vi "WSVCAP SHL Host LL Interface Core.vi"(0 "Message In":string, 11 "error in":errorcluster, 12 "Log (T)":bool=TRUE, 13 "Function":T5, 14 "FPGA":T1) -> (3 "System":T2={"Settings"={"I2C Slave Address"=144, "I2C Clock Rate (Hz)"=20.0, "SRL Clock Rate (Hz)"=50000.0, "Simulate FPGA"=TRUE, "C1 Cap DAC Default"=165, "C2 Cap DAC Default"=165, "C3 Cap DAC Default"=134, "C4 Cap DAC Default"=150, "DAC Out Vref (V)"=0.0}, "FPGA Resource"="", "Online"=FALSE, "I2C Wait Ticks"=0, "SRL Wait Ticks"=0, "FPGA VI Reference (FPGA Mode)"=refnum, "FPGA VI Reference (Sim Mode)"=refnum} {"Settings"."DAC Out Vref (V)" format="%.3f V"; "Settings"."C4 Cap DAC Default" format="0x%02x"; "Settings"."C3 Cap DAC Default" format="0x%02x"; "Settings"."C2 Cap DAC Default" format="0x%02x"; "Settings"."C1 Cap DAC Default" format="0x%02x"; "Settings"."SRL Clock Rate (Hz)" format="%.0f Hz"; "Settings"."I2C Clock Rate (Hz)" format="%.0f Hz"; "Settings"."I2C Slave Address" format="0x%02x"}, 4 "Message Out":string, 15 "error out":errorcluster)   [LabVIEW 2017]
uses:
  Type Defs/WSVCAP SHL Function Enum.ctl
  Type Defs/WSVCAP SHL Core System Cluster.ctl
  Type Defs/WSVCAP SHL I2C Settings Cluster.ctl
  Type Defs/WSVCAP SHL FPGA Ref.ctl
  Type Defs/WSVCAP SHL FPGA Enum.ctl
  user.lib/Utilities/Type Defs/MISC IO Choice Enum.ctl
  Type Defs/WSVCAP SHL Gatekeeper Operation Enum.ctl
  user.lib/Configuration Files/Type Defs/CFG File Operation Enum.ctl
  Type Defs/WSVCAP SHL Top Level Control Enum.ctl
  <vilib>/FPGAPlugInAG/PXI-7813R/niLvFpga_Open_PXI-7813R.vi
  <vilib>/FPGAPlugInAG/PXI-7813R/niLvFpga_Reset_PXI-7813R.vi
  <vilib>/FPGAPlugInAG/PXI-7813R/niLvFpga_Run_PXI-7813R.vi
  <vilib>/FPGAPlugInAG/PXI-7813R/niLvFpga_Abort_PXI-7813R.vi
  <vilib>/FPGAPlugInAG/PXI-7813R/niLvFpga_Close_PXI-7813R.vi
  <vilib>/rvi/interface/nirviOpenFPGA/nirviOpenFPGA.xnode
  FPGA Bitfiles/WSVCAPShell_WiSpryFPGA1_WSVCAPSHLFPGATLT_ffr+nD2N+rA.lvbitx
  <vilib>/rvi/interface/nirviMethod/nirviMethod.xnode
  <vilib>/rvi/interface/nirviCloseFPGA/nirviCloseFPGA.xnode
  Host SRL/Host SRL.lvlib
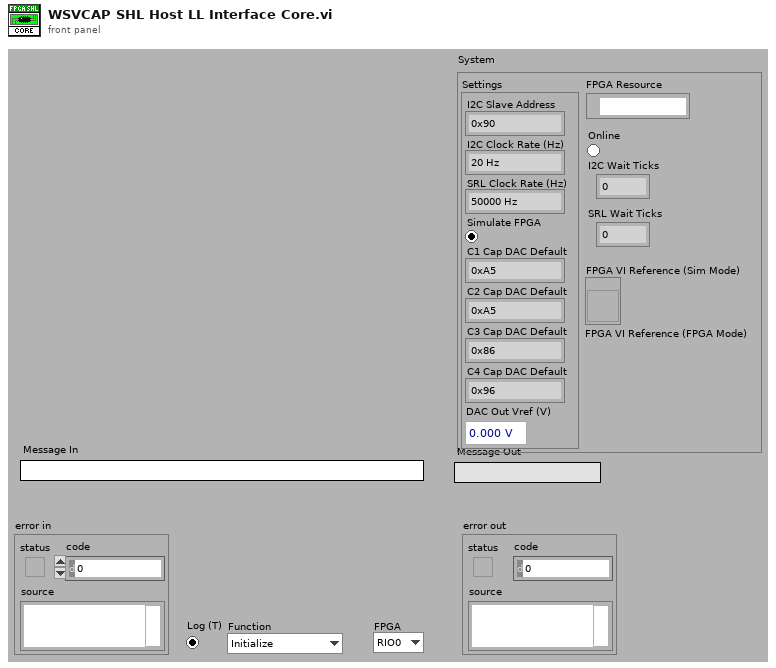
[diagram p1: front panel]
types:
  T1 = typedef "WSVCAP SHL FPGA Enum.ctl" = enum16{"RIO0", "RIO1"}
  T2 = typedef "WSVCAP SHL Core System Cluster.ctl" = cluster{"Settings":T3, "FPGA Resource":tag, "Online":bool, "I2C Wait Ticks":u32, "SRL Wait Ticks":u32, "FPGA VI Reference (FPGA Mode)":T4, "FPGA VI Reference (Sim Mode)":refnum<vi>}
  T3 = typedef "WSVCAP SHL I2C Settings Cluster.ctl" = cluster{"I2C Slave Address":u8, "I2C Clock Rate (Hz)":dbl, "SRL Clock Rate (Hz)":dbl, "Simulate FPGA":bool, "C1 Cap DAC Default":u8, "C2 Cap DAC Default":u8, "C3 Cap DAC Default":u8, "C4 Cap DAC Default":u8, "DAC Out Vref (V)":dbl}
  T4 = typedef "WSVCAP SHL FPGA Ref.ctl" = refnum<k20>
  T5 = typedef "WSVCAP SHL Function Enum.ctl" = enum16{"Initialize", "Configure I2C", "Configure SRL", "Write I2C", "Read I2C", "Write SRL", "Start SRL Cycle", "Stop SRL Cycle", "Get Status", "Close"}
  T6 = typedef "WSVCAP SHL Gatekeeper Operation Enum.ctl" = enum16{"Initialize", "Lock", "Unlock", "Close"}
  T7 = typedef "MISC IO Choice Enum.ctl" = enum16{"Read", "Write"}
  T8 = typedef "CFG File Operation Enum.ctl" = enum16{"Read", "Write", "Copy", "Edit"}
  T9 = enum32{"Invalid", "Standard", "Closed", "Hidden", "Minimized", "Maximized"}
  T10 = typedef "WSVCAP SHL Top Level Control Enum.ctl" = enum16{"Start", "Cmd", "Transaction", "Wait Ticks", "Socket Mask", "UUT Set", "Slave Address", "Sub Address", "Bytes to Write", "Bytes to Read", "Write Data", "Write Flag", "Read Data", "Read Flag", "Ack Read", "Read Status Flag", "Ack Read Status", "Status", "Cycle Count", "Stop Cycle", "Exit"}
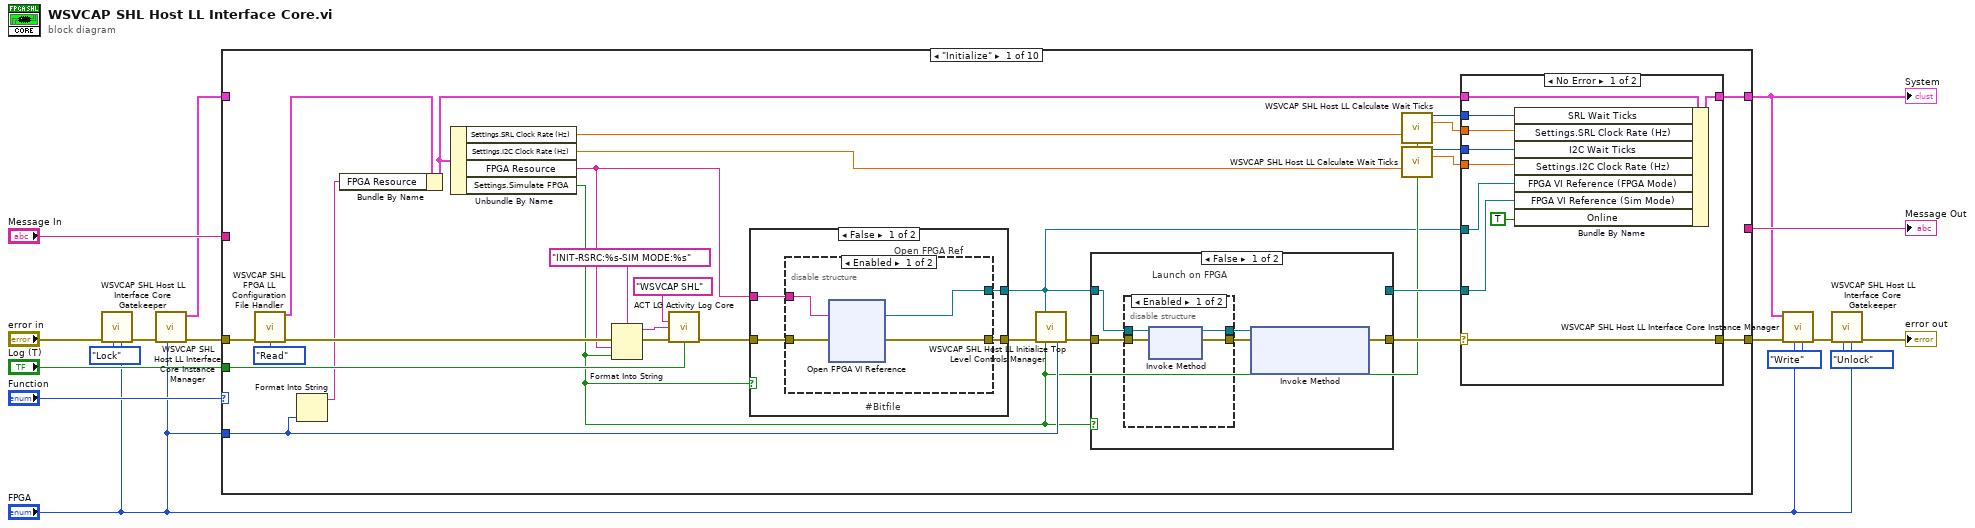
[diagram p0: block diagram]
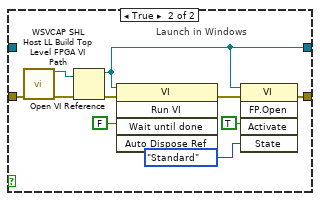
[diagram p5: hidden frame]
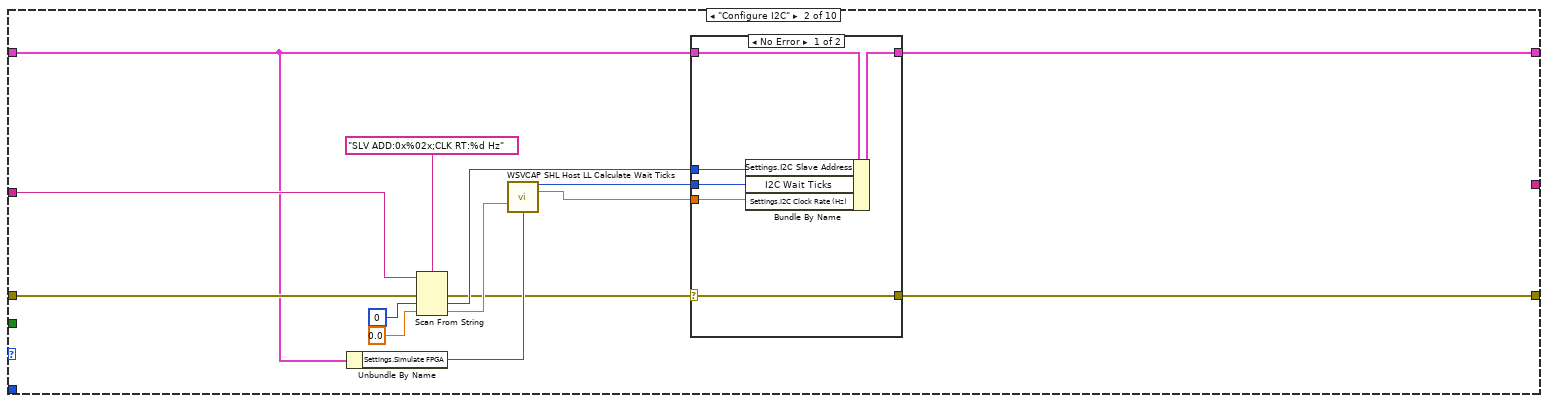
[diagram p7: hidden frame]
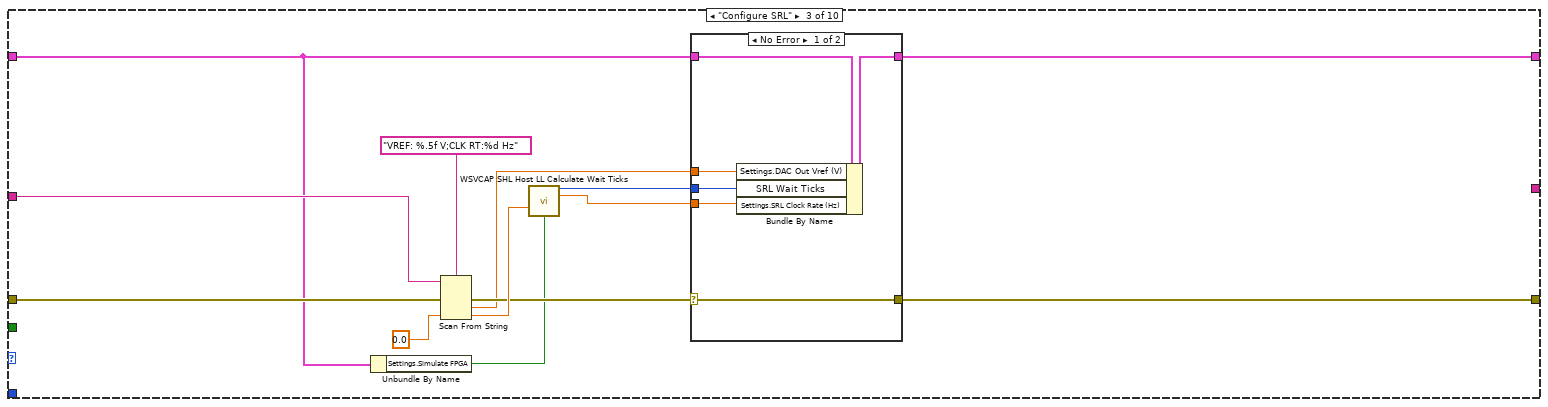
[diagram p9: hidden frame]
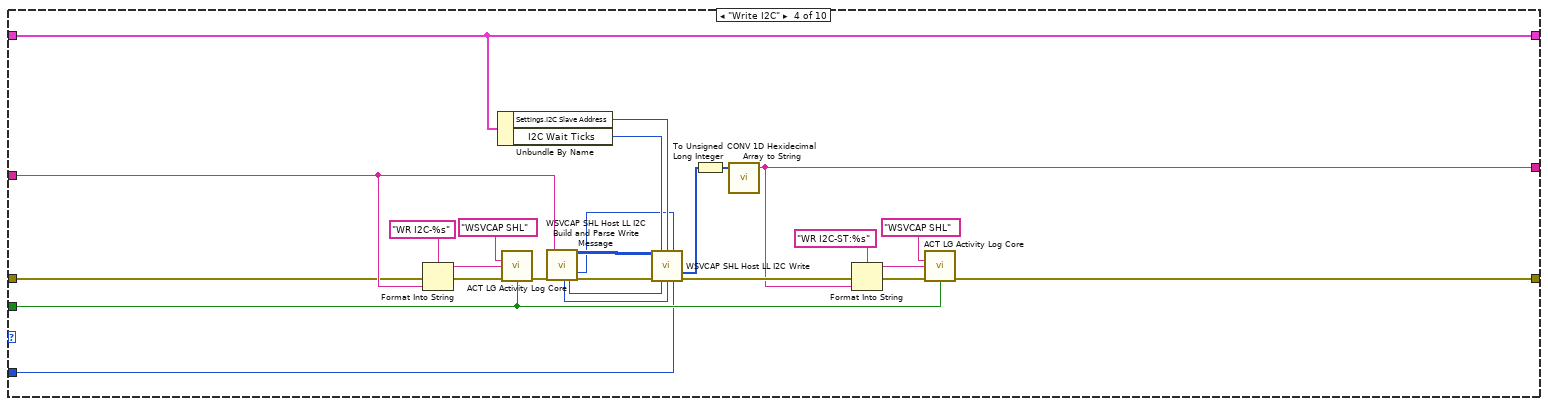
[diagram p11: hidden frame]
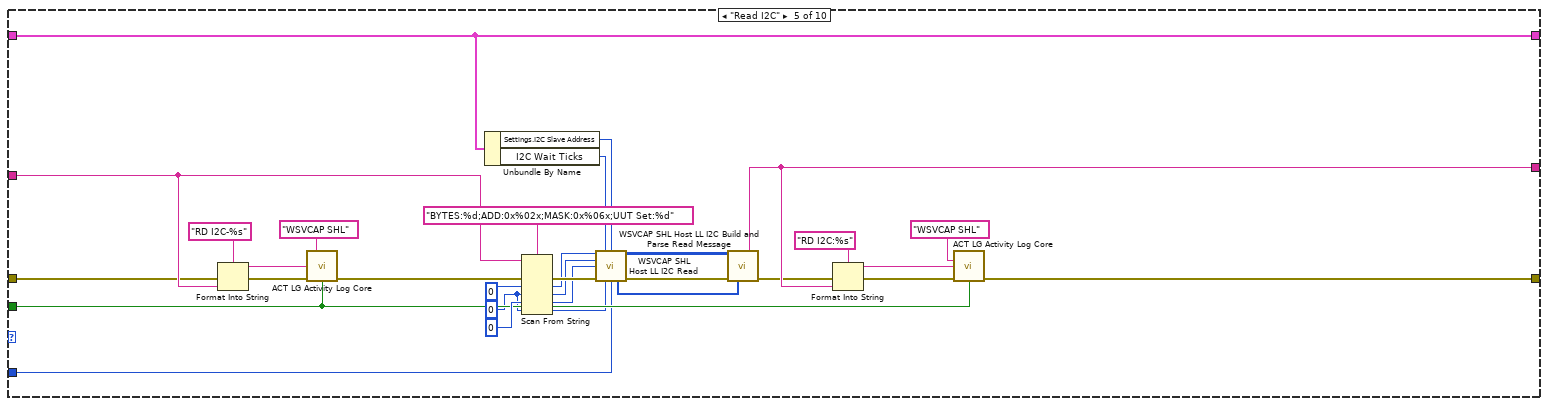
[diagram p12: hidden frame]
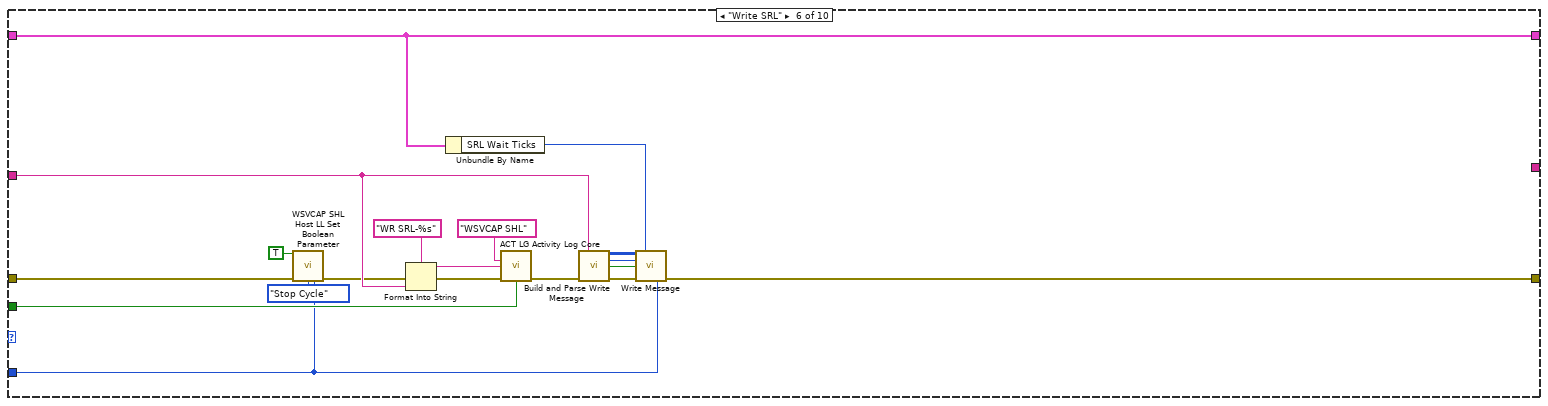
[diagram p13: hidden frame]
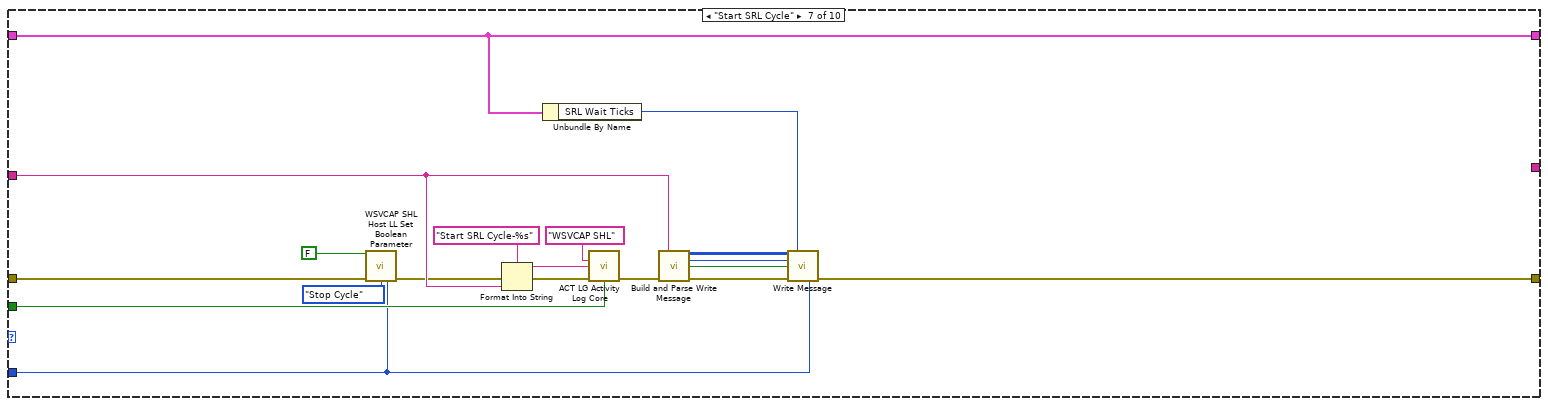
[diagram p14: hidden frame]
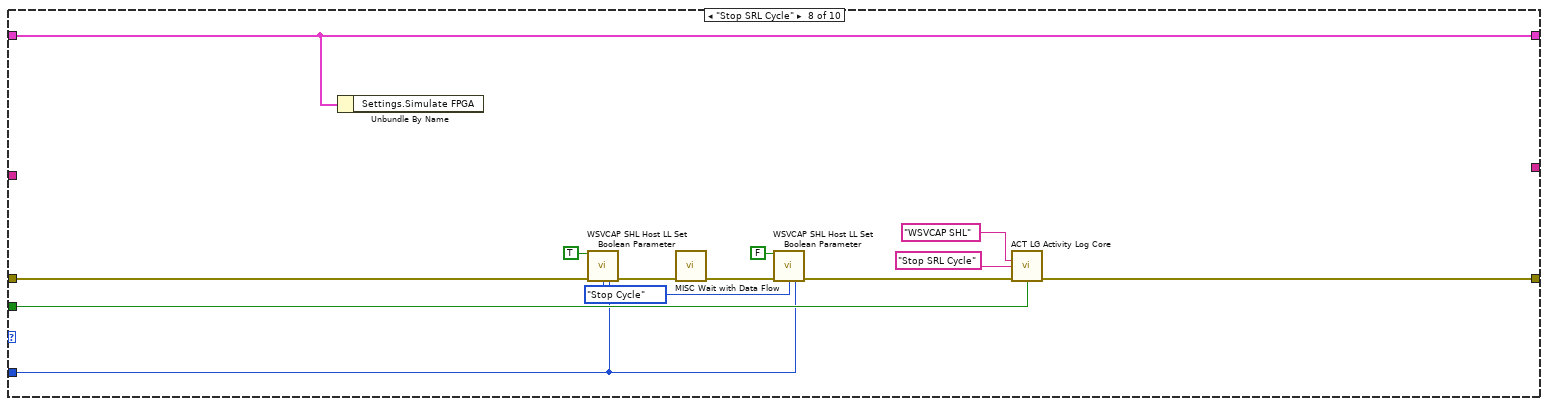
[diagram p15: hidden frame]
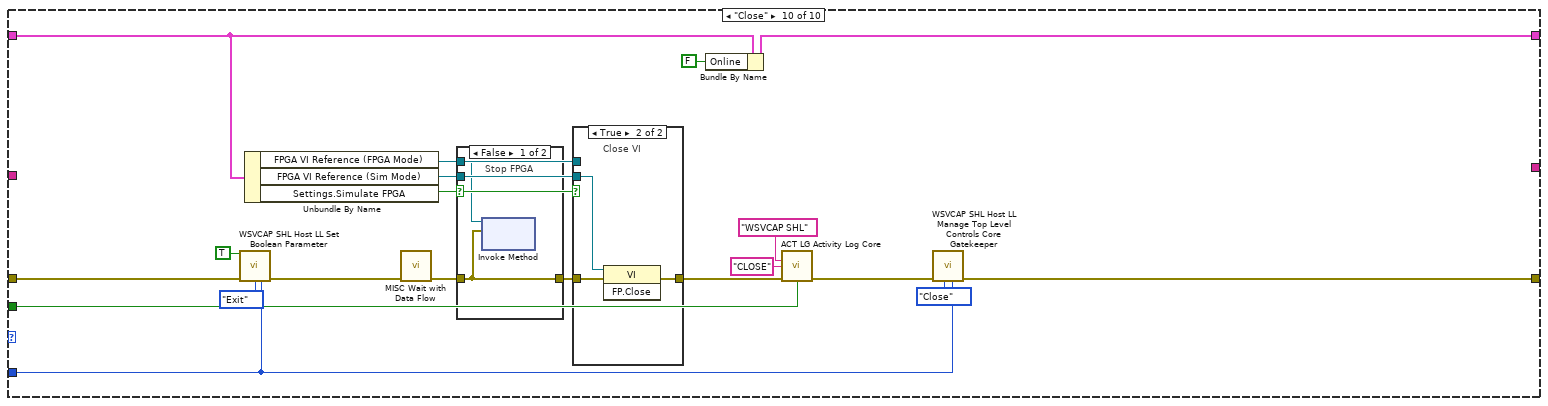
[diagram p17: hidden frame]
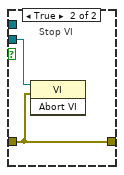
[diagram p18: hidden frame]
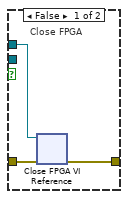
[diagram p19: hidden frame]
diagram:
  n1 = call "WSVCAP SHL Host LL Interface Core Gatekeeper.vi"("FPGA"="FPGA", "Operation"=WSVCAP_SHL_Gatekeeper_Operation_Enum."Lock", "error in (no error)"="error in") -> ("error out"=w4:errorcluster)  [unwired: 8 in]
  n2 = call "WSVCAP SHL Host LL Interface Core Instance Manager.vi"("FPGA"="FPGA", "error in (no error)"=w4) -> ("error out"=w10:errorcluster, "FGPA Interface Out"=w9:T2)  [unwired: 8 in]
  n3 = case shown="\"Initialize\"" "Function" {
    tunnel: w10 -> [w40 w99 w120 w149 w170 w196 w210 w234 w239 w257]
    tunnel: "Message In" -> [_ w98 w119 w150 w171 w199 w218 _ _ _]
    tunnel: [w43 w100 w121 w151 w167 w191 w216 w237 w239 w242] -> w12
    tunnel: [w44 w101 w122 w137 w163 w193 w214 w226 w240 w260] -> w11
    tunnel: w9 -> [_ w94 w117 w137 w163 w193 w214 w226 w240 w250]
    tunnel: [_ _ _ w141 w172 _ _ _ _ _] -> w14
    tunnel: "Log (T)" -> [w33 _ _ w138 w164 w198 w217 w236 _ w253]
    tunnel: "FPGA" -> [w21 _ _ w132 w158 w190 w208 w232 _ w241]
    frame "Initialize" {
      n4 = call "WSVCAP SHL FPGA LL Configuration File Handler.vi"("Error In (no error)"=w40, "Operation"=CFG_File_Operation_Enum."Read") -> ("Object Cluster Out"=w23:T2, "Error Out"=w38:errorcluster)  [unwired: 11 in, 1 out]
      n5 = Format Into String(w21) -> (resulting string=w24:string)  [unwired: 3 in, 1 out]
      n6 = Bundle By Name(cluster=w23, "FPGA Resource"=w24) -> (w22:T2)
      n7 = Unbundle By Name(w22) -> ("Settings.SRL Clock Rate (Hz)"=w31:dbl, "Settings.I2C Clock Rate (Hz)"=w35:dbl, "FPGA Resource"=w28:tag, "Settings.Simulate FPGA"=w20:bool)
      n8 = Format Into String(format string="INIT-RSRC:%s-SIM MODE:%s", error in=w38, w28, w20) -> (resulting string=w39:string, error out=w37:errorcluster)  [unwired: 1 in]
      n9 = call "ACT LG Activity Log Core.vi"("Source"="WSVCAP SHL", "Log Line"=w39, "Error In (no error)"=w37, "Log (T)"=w33) -> ("Error Out"=w27:errorcluster)  [unwired: 10 in, 1 out]
      n10 = case shown="False" w20 {
        tunnel: [w48 w54] -> w19
        tunnel: w27 -> [w47 w54]
        tunnel: [w46 _] -> w17
        tunnel: w28 -> [w45 _]
        frame False {
          # "#Bitfile"
          # "Open FPGA Ref"
          n11 = disable-structure shown="Enabled" {
            disable-tunnel: w47 -> [w52 w53]
            disable-tunnel: [w51 w53] -> w48
            disable-tunnel: [w50 _] -> w46
            disable-tunnel: w45 -> [w49 _]
            frame Enabled {
              n12 = xnode "Open FPGA VI Reference"("error in"=w52, "resource name"=w49) -> ("FPGA VI Reference Out"=w50:T4, "error out"=w51:errorcluster)
            }
            frame Disabled {
            }
          }
        }
        frame True {
          # "Simulate FPGA"
        }
      }
      n13 = call "WSVCAP SHL Host LL Initialize Top Level Controls Manager.vi"("FPGA VI Reference (Init Only)"=w17, "error in (no error)"=w19, "Simulate FPGA (Init Only)"=w20, "FPGA"=w21) -> ("error out"=w18:errorcluster)  [unwired: 11 in]
      n14 = case shown="False" w20 {
        tunnel: w18 -> [w58 w68]
        tunnel: [w57 w71] -> w26
        tunnel: w17 -> [w55 _]
        tunnel: [_ w72] -> w25
        frame False {
          # "Launch on FPGA"
          n15 = disable-structure shown="Enabled" {
            disable-tunnel: [w63 w65] -> w59
            disable-tunnel: w58 -> [w62 w65]
            disable-tunnel: [w61 w64] -> w56
            disable-tunnel: w55 -> [w60 w64]
            frame Enabled {
              n16 = xnode "Invoke Method"("FPGA VI Reference In"=w60, "error in"=w62) -> ("FPGA VI Reference Out"=w61:T4, "error out"=w63:errorcluster)
            }
            frame Disabled {
            }
          }
          n17 = xnode "Invoke Method"("FPGA VI Reference In"=w56, "error in"=w59) -> ("error out"=w57:errorcluster)  [unwired: 1 in, 1 out]
        }
        frame True {
          # "Launch in Windows"
          n18 = call "WSVCAP SHL Host LL Build Top Level FPGA VI Path.vi"("Error In (no error)"=w68) -> ("Top Level FPGA VI Path"=w66:path, "Error Out"=w67:errorcluster)  [unwired: 13 in]
          n19 = Open VI Reference(vi path=w66, error in (no error)=w67) -> (vi reference=w72:refnum<vi>, error out=w75:errorcluster)  [unwired: 4 in]
          n20 = invoke class="VI" method="Run VI"(reference=w72, error in=w75, "Wait until done"=FALSE ("Wait Until Done")) -> (error out=w73:errorcluster)  [unwired: 2 in, 4 out]
          n21 = invoke class="VI" method="FP.Open"(reference=w72, error in=w73, "Activate"=TRUE ("Activate?"), "State"=T9."Standard" ("Front Panel Window:State")) -> (error out=w71:errorcluster)  [unwired: 1 in, 4 out]
        }
      }
      n22 = call "WSVCAP SHL Host LL Calculate Wait Ticks.vi"("Clock Rate (Hz)"=w31, "Simulate FPGA"=w20) -> ("Wait Ticks"=w30:u32, "Actual Rate (Hz)"=w29:dbl)  [unwired: 12 in]
      n23 = call "WSVCAP SHL Host LL Calculate Wait Ticks.vi"("Clock Rate (Hz)"=w35, "Simulate FPGA"=w20) -> ("Wait Ticks"=w32:u32, "Actual Rate (Hz)"=w42:dbl)  [unwired: 12 in]
      n24 = case shown="No Error" w26 {
        selector: w26 -> [w83 w86]
        tunnel: w22 -> [w85 w87]
        tunnel: [w84 w87] -> w44
        tunnel: [w83 w86] -> w43
        tunnel: w42 -> [w82 _]
        tunnel: w32 -> [w81 _]
        tunnel: w30 -> [w80 _]
        tunnel: w29 -> [w79 _]
        tunnel: w17 -> [w77 _]
        tunnel: w25 -> [w76 _]
        frame No Error {
          n25 = Bundle By Name(cluster=w85, "SRL Wait Ticks"=w80, "Settings.SRL Clock Rate (Hz)"=w79, "I2C Wait Ticks"=w81, "Settings.I2C Clock Rate (Hz)"=w82, "FPGA VI Reference (FPGA Mode)"=w77, "FPGA VI Reference (Sim Mode)"=w76, "Online"=TRUE) -> (w84:T2)
        }
        frame Error {
        }
      }
    }
    frame "Configure I2C" {
      n26 = Unbundle By Name(w94) -> ("Settings.Simulate FPGA"=w93:bool)
      n27 = Scan From String(format string="SLV ADD:0x%02x;CLK RT:%d Hz", input string=w98, error in=w99, default 1=u8 0 ("I2C_Slave Address"), default 2=0.0 ("Clock Rate (Hz)")) -> (error out=w88:errorcluster, output 1=w95:u8, output 2=w91:dbl)  [unwired: 1 in, 2 out]
      n28 = call "WSVCAP SHL Host LL Calculate Wait Ticks.vi"("Clock Rate (Hz)"=w91, "Simulate FPGA"=w93) -> ("Wait Ticks"=w89:u32, "Actual Rate (Hz)"=w90:dbl)  [unwired: 12 in]
      n29 = case shown="No Error" w88 {
        selector: w88 -> [w105 w108]
        tunnel: w94 -> [w107 w109]
        tunnel: [w106 w109] -> w101
        tunnel: [w105 w108] -> w100
        tunnel: w95 -> [w104 _]
        tunnel: w90 -> [w103 _]
        tunnel: w89 -> [w102 _]
        frame No Error {
          n30 = Bundle By Name(cluster=w107, "Settings.I2C Slave Address"=w104, "I2C Wait Ticks"=w102, "Settings.I2C Clock Rate (Hz)"=w103) -> (w106:T2)
        }
        frame Error {
        }
      }
    }
    frame "Configure SRL" {
      n31 = Unbundle By Name(w117) -> ("Settings.Simulate FPGA"=w111:bool)
      n32 = Scan From String(format string="VREF: %.5f V;CLK RT:%d Hz", input string=w119, error in=w120, default 2=0.0 ("Clock Rate (Hz)")) -> (error out=w112:errorcluster, output 1=w110:dbl, output 2=w115:dbl)  [unwired: 2 in, 2 out]
      n33 = call "WSVCAP SHL Host LL Calculate Wait Ticks.vi"("Clock Rate (Hz)"=w115, "Simulate FPGA"=w111) -> ("Wait Ticks"=w114:u32, "Actual Rate (Hz)"=w113:dbl)  [unwired: 12 in]
      n34 = case shown="No Error" w112 {
        selector: w112 -> [w126 w129]
        tunnel: w117 -> [w128 w130]
        tunnel: [w127 w130] -> w122
        tunnel: [w126 w129] -> w121
        tunnel: w113 -> [w125 _]
        tunnel: w114 -> [w124 _]
        tunnel: w110 -> [w123 _]
        frame No Error {
          n35 = Bundle By Name(cluster=w128, "Settings.DAC Out Vref (V)"=w123, "SRL Wait Ticks"=w124, "Settings.SRL Clock Rate (Hz)"=w125) -> (w127:T2)
        }
        frame Error {
        }
      }
    }
    frame "Write I2C" {
      n36 = Format Into String(format string="WR I2C-%s", error in=w149, w150) -> (resulting string=w146:string, error out=w148:errorcluster)  [unwired: 1 in]
      n37 = Unbundle By Name(w137) -> ("Settings.I2C Slave Address"=w134:u8, "I2C Wait Ticks"=w136:u32)
      n38 = call "ACT LG Activity Log Core.vi"("Source"="WSVCAP SHL", "Log Line"=w146, "Error In (no error)"=w148, "Log (T)"=w138) -> ("Error Out"=w153:errorcluster)  [unwired: 10 in, 1 out]
      n39 = call "WSVCAP SHL Host LL I2C Build and Parse Write Message.vi"("error in"=w153, "Message In"=w150) -> ("UUT Set (0/1) Out (Legacy)"=w133:u8, "Sub Address Out"=w135:u8, "C Write Data Out [DUT Ordered]"=w155:u8[][], "Socket Mask [U64] Out"=w131:u64, "error out"=w156:errorcluster)  [unwired: 12 in, 1 out]
      n40 = call "WSVCAP SHL Host LL I2C Write.vi"("C1 Data Out [DUT Ordered]"=w155, "Wait Ticks"=w136, "Slave Address"=w134, "Socket Mask [U64]"=w131, "error in"=w156, "Sub Address"=w135, "UUT Set (0/1)"=w133, "FPGA"=w132) -> ("Status"=w143:u8[], "error out"=w145:errorcluster)  [unwired: 6 in]
      n41 = To Unsigned Long Integer(number=w143) -> (unsigned 32bit integer=w142:u32[])
      n42 = call "CONV 1D Hexidecimal Array to String.vi"("1-D Hexidecimal"=w142) -> ("String"=w141:string)  [unwired: 8 in]
      n43 = Format Into String(format string="WR I2C-ST:%s", error in=w145, w141) -> (resulting string=w139:string, error out=w144:errorcluster)  [unwired: 1 in]
      n44 = call "ACT LG Activity Log Core.vi"("Source"="WSVCAP SHL", "Log Line"=w139, "Error In (no error)"=w144, "Log (T)"=w138) -> ("Error Out"=w151:errorcluster)  [unwired: 10 in, 1 out]
    }
    frame "Read I2C" {
      w160 = u8 0 ("Sub Address [U8]")
      n45 = Format Into String(format string="RD I2C-%s", error in=w170, w171) -> (resulting string=w176:string, error out=w178:errorcluster)  [unwired: 1 in]
      n46 = call "ACT LG Activity Log Core.vi"("Source"="WSVCAP SHL", "Log Line"=w176, "Error In (no error)"=w178, "Log (T)"=w164) -> ("Error Out"=w169:errorcluster)  [unwired: 10 in, 1 out]
      n47 = Unbundle By Name(w163) -> ("Settings.I2C Slave Address"=w161:u8, "I2C Wait Ticks"=w162:u32)
      n48 = Scan From String(format string="BYTES:%d;ADD:0x%02x;MASK:0x%06x;UUT Set:%d", input string=w171, error in=w169, default 1=u8 0 ("Bytes to Read"), default 2=w160, default 3=u64 0 ("Socket Mask [U32]"), default 4=w160) -> (error out=w187:errorcluster, output 1=w184:u8, output 2=w182:u8, output 3=w183:u64, output 4=w159:u8)  [unwired: 1 in, 2 out]
      n49 = call "WSVCAP SHL Host LL I2C Read.vi"("Bytes to Read"=w184, "Wait Ticks"=w162, "Slave Address"=w161, "Sub Address [U8]"=w182, "Socket Mask [U64]"=w183, "error in"=w187, "UUT Set (0/1)"=w159, "FPGA"=w158) -> ("Cap1:24 Read Data"=w180:u8[][], "Status"=w157:u8[], "error out"=w181:errorcluster)  [unwired: 5 in]
      n50 = call "WSVCAP SHL Host LL I2C Build and Parse Read Message.vi"("C1 Read Data In"=w180, "error in"=w181, "Status In"=w157) -> ("Message Out"=w172:string, "error out"=w168:errorcluster)  [unwired: 9 in, 2 out]
      n51 = Format Into String(format string="RD I2C:%s", error in=w168, w172) -> (resulting string=w173:string, error out=w175:errorcluster)  [unwired: 1 in]
      n52 = call "ACT LG Activity Log Core.vi"("Source"="WSVCAP SHL", "Log Line"=w173, "Error In (no error)"=w175, "Log (T)"=w164) -> ("Error Out"=w167:errorcluster)  [unwired: 10 in, 1 out]
    }
    frame "Write SRL" {
      n53 = call "WSVCAP SHL Host LL Set Boolean Parameter.vi"("Boolean In"=TRUE ("Cycle (F:Write/Read - T:Write Only - No Read)"), "error in (no error)"=w196, "FPGA Top Level Control"=WSVCAP_SHL_Top_Level_Control_Enum."Stop Cycle", "FPGA"=w190) -> ("error out"=w195:errorcluster)  [unwired: 11 in]
      n54 = Format Into String(format string="WR SRL-%s", error in=w195, w199) -> (resulting string=w201:string, error out=w203:errorcluster)  [unwired: 1 in]
      n55 = Unbundle By Name(w193) -> ("SRL Wait Ticks"=w192:u32)
      n56 = call "ACT LG Activity Log Core.vi"("Source"="WSVCAP SHL", "Log Line"=w201, "Error In (no error)"=w203, "Log (T)"=w198) -> ("Error Out"=w200:errorcluster)  [unwired: 10 in, 1 out]
      n57 = call "Build and Parse Write Message.vi"("Message In"=w199, "error in"=w200) -> ("Write Data Out [DUT Ordered]"=w205:u8[][], "Socket Mask [U32] Out"=w194:u32, "Cycle Mode Out"=w188:bool, "error out"=w206:errorcluster)  [unwired: 8 in, 2 out]
      n58 = call "Write Message.vi"("SRL Data"=w205, "Wait Ticks"=w192, "Socket Mask"=w194, "Cycle Mode"=w188, "error in"=w206, "FPGA"=w190) -> ("error out"=w191:errorcluster)  [unwired: 8 in, 1 out]
    }
    frame "Start SRL Cycle" {
      n59 = call "WSVCAP SHL Host LL Set Boolean Parameter.vi"("Boolean In"=FALSE ("Cycle (F:Write/Read - T:Write Only - No Read)"), "error in (no error)"=w210, "FPGA Top Level Control"=WSVCAP_SHL_Top_Level_Control_Enum."Stop Cycle", "FPGA"=w208) -> ("error out"=w209:errorcluster)  [unwired: 11 in]
      n60 = Format Into String(format string="Start SRL Cycle-%s", error in=w209, w218) -> (resulting string=w220:string, error out=w222:errorcluster)  [unwired: 1 in]
      n61 = Unbundle By Name(w214) -> ("SRL Wait Ticks"=w213:u32)
      n62 = call "ACT LG Activity Log Core.vi"("Source"="WSVCAP SHL", "Log Line"=w220, "Error In (no error)"=w222, "Log (T)"=w217) -> ("Error Out"=w219:errorcluster)  [unwired: 10 in, 1 out]
      n63 = call "Build and Parse Write Message.vi"("Message In"=w218, "error in"=w219) -> ("Write Data Out [DUT Ordered]"=w224:u8[][], "Socket Mask [U32] Out"=w215:u32, "Cycle Mode Out"=w207:bool, "error out"=w225:errorcluster)  [unwired: 8 in, 2 out]
      n64 = call "Write Message.vi"("SRL Data"=w224, "Wait Ticks"=w213, "Socket Mask"=w215, "Cycle Mode"=w207, "error in"=w225, "FPGA"=w208) -> ("error out"=w216:errorcluster)  [unwired: 8 in, 1 out]
    }
    frame "Stop SRL Cycle" {
      w231 = WSVCAP_SHL_Top_Level_Control_Enum."Stop Cycle" ("FPGA Top Level Control")
      n65 = Unbundle By Name(w226) -> ()  [unwired: 1 out]
      n66 = call "WSVCAP SHL Host LL Set Boolean Parameter.vi"("Boolean In"=TRUE ("Cycle (F:Write/Read - T:Write Only - No Read)"), "error in (no error)"=w234, "FPGA Top Level Control"=w231, "FPGA"=w232) -> ("error out"=w230:errorcluster)  [unwired: 11 in]
      n67 = call "MISC Wait with Data Flow.vi"("Error In (no error)"=w230) -> ("Error Out"=w229:errorcluster)  [unwired: 8 in, 2 out]
      n68 = call "WSVCAP SHL Host LL Set Boolean Parameter.vi"("Boolean In"=FALSE ("Cycle (F:Write/Read - T:Write Only - No Read)"), "error in (no error)"=w229, "FPGA Top Level Control"=w231, "FPGA"=w232) -> ("error out"=w233:errorcluster)  [unwired: 11 in]
      n69 = call "ACT LG Activity Log Core.vi"("Source"="WSVCAP SHL", "Log Line"="Stop SRL Cycle" ("format string"), "Error In (no error)"=w233, "Log (T)"=w236) -> ("Error Out"=w237:errorcluster)  [unwired: 10 in, 1 out]
    }
    frame "Get Status" {
    }
    frame "Close" {
      n70 = call "WSVCAP SHL Host LL Set Boolean Parameter.vi"("Boolean In"=TRUE ("Start"), "error in (no error)"=w257, "FPGA Top Level Control"=WSVCAP_SHL_Top_Level_Control_Enum."Exit", "FPGA"=w241) -> ("error out"=w246:errorcluster)  [unwired: 11 in]
      n71 = Unbundle By Name(w250) -> ("FPGA VI Reference (FPGA Mode)"=w249:T4, "FPGA VI Reference (Sim Mode)"=w248:refnum<vi>, "Settings.Simulate FPGA"=w247:bool)
      n72 = call "MISC Wait with Data Flow.vi"("Error In (no error)"=w246) -> ("Error Out"=w251:errorcluster)  [unwired: 8 in, 2 out]
      n73 = case shown="False" w247 {
        tunnel: w249 -> [w262 _]
        tunnel: w251 -> [w261 w263]
        tunnel: [w261 w263] -> w252
        tunnel: w248 -> [_ w264]
        frame False {
          # "Stop FPGA"
          n74 = xnode "Invoke Method"("FPGA VI Reference In"=w262, "error in"=w261) -> ()  [unwired: 2 out]
        }
        frame True {
          # "Stop VI"
          n75 = invoke class="VI" method="Abort VI"(reference=w264, error in=w263) -> ()  [unwired: 1 in, 3 out]
        }
      }
      n76 = case shown="True" w247 {
        tunnel: w252 -> [w267 w270]
        tunnel: w249 -> [w266 _]
        tunnel: [w265 w269] -> w245
        tunnel: w248 -> [_ w268]
        frame False {
          # "Close FPGA"
          n77 = xnode "Close FPGA VI Reference"("FPGA VI Reference In"=w266, "error in"=w267) -> ("error out"=w265:errorcluster)
        }
        frame True {
          # "Close VI"
          n78 = invoke class="VI" method="FP.Close"(reference=w268, error in=w270) -> (error out=w269:errorcluster)  [unwired: 1 in, 2 out]
        }
      }
      n79 = Bundle By Name(cluster=w250, "Online"=FALSE) -> (w260:T2)
      n80 = call "ACT LG Activity Log Core.vi"("Source"="WSVCAP SHL", "Log Line"="CLOSE", "Error In (no error)"=w245, "Log (T)"=w253) -> ("Error Out"=w243:errorcluster)  [unwired: 10 in, 1 out]
      n81 = call "WSVCAP SHL Host LL Manage Top Level Controls Core Gatekeeper.vi"("FPGA"=w241, "Operation"=WSVCAP_SHL_Gatekeeper_Operation_Enum."Close", "error in (no error)"=w243) -> ("error out"=w242:errorcluster)  [unwired: 8 in]
    }
  }
  "Message Out" <- w14
  "System" <- w11
  n82 = call "WSVCAP SHL Host LL Interface Core Instance Manager.vi"("I/O Choice (read)"=MISC_IO_Choice_Enum."Write", "FPGA"="FPGA", "error in (no error)"=w12, "FPGA Interface In"=w11) -> ("error out"=w7:errorcluster)  [unwired: 6 in, 1 out]
  n83 = call "WSVCAP SHL Host LL Interface Core Gatekeeper.vi"("FPGA"="FPGA", "Operation"=WSVCAP_SHL_Gatekeeper_Operation_Enum."Unlock", "error in (no error)"=w7) -> ("error out"=→"error out":errorcluster)  [unwired: 8 in]
